vi "UtilityLib.time 2 string.vi"(1 "time":dbl[](array[numeric])) -> (0 "timeString":string[](array[string]))   [LabVIEW 2014, in "UtilityLib.lvlib"]
doc: "Converts a time in seconds to a string in format \"HHHH:MM:SS\""
uses:
  UtilityLib.lvlib
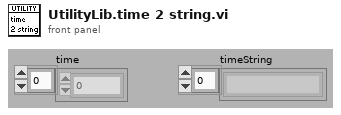
[diagram p1: front panel]
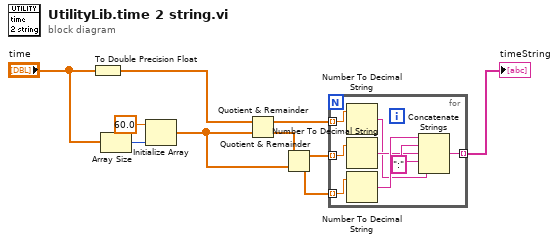
[diagram p0: block diagram]
diagram:
  n1 = To Double Precision Float(number="time") -> (double precision float=w5:dbl[])
  n2 = Array Size(array="time") -> (size(s)=w8:i32)
  n3 = Initialize Array(60.0 ("element"), w8) -> (w10:dbl[])
  n4 = Quotient & Remainder(x=w5, y=w10) -> (x-y*floor(x/y)=w1:dbl[], floor(x/y)=w2:dbl[])
  n5 = Quotient & Remainder(x=w2, y=w10) -> (x-y*floor(x/y)=w4:dbl[], floor(x/y)=w3:dbl[])
  n6 = for {
    tunnel: w1 -> [w18] mode=indexing
    tunnel: w4 -> [w17] mode=indexing
    tunnel: w3 -> [w16] mode=indexing
    tunnel: [w11] -> w6 mode=indexing
    w14 = ":"
    n7 = Number To Decimal String(number=w18) -> (decimal integer string=w12:string)  [unwired: 1 in]
    n8 = Number To Decimal String(number=w17) -> (decimal integer string=w13:string)  [unwired: 1 in]
    n9 = Number To Decimal String(number=w16) -> (decimal integer string=w15:string)  [unwired: 1 in]
    n10 = Concatenate Strings(w15, w14, w13, w14, w12) -> (w11:string)
  }
  "timeString" <- w6
